vi "Read_Battery_Clear_Fault_VI.vi"() -> ()   [LabVIEW 2017]
uses:
  <vilib>/Plasmionique/MB Master/MB_Master_TCP/MB_Master_TCP.lvclass
  C:/Program Files (x86)/National Instruments/LabVIEW 2017/vi.lib/Plasmionique/MB Master/MB_Master/MB_Master.lvclass
  <vilib>/Plasmionique/MB Master/MB Master.lvlib
panel:
  out "Error?":string
  out "BMS IP Address":string
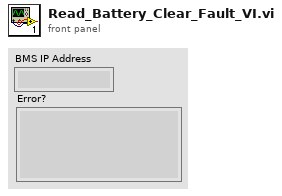
[diagram p1: front panel]
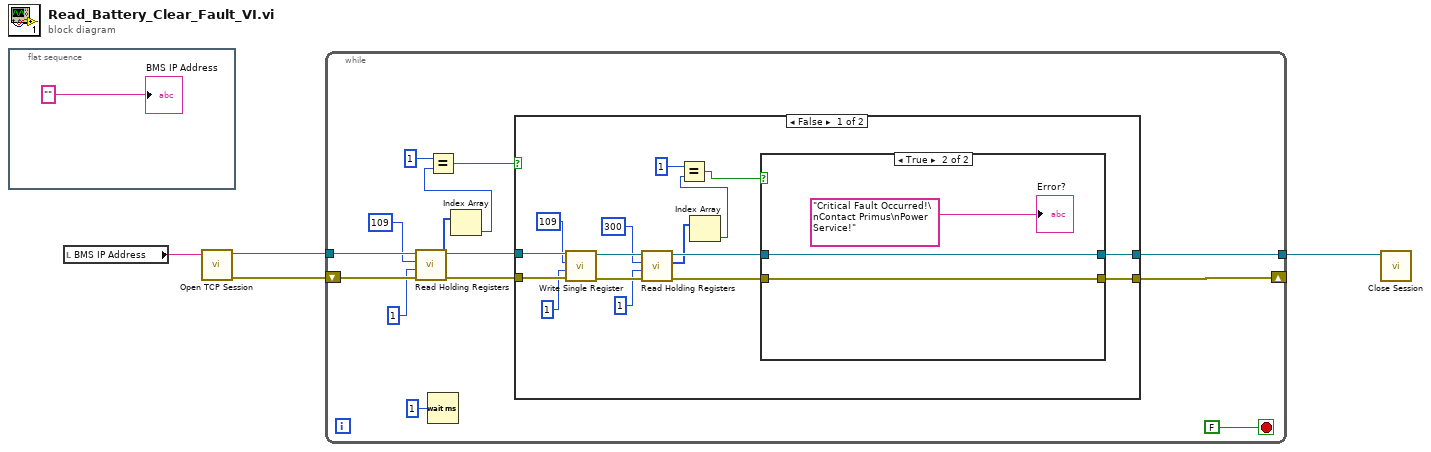
[diagram p0: block diagram]
diagram:
  n1 = flat-sequence {
    frame #0 {
      "BMS IP Address" <- ""
    }
  }
  n2 = local read "BMS IP Address"() -> (w2:string)
  n3 = call <vilib>:"Open TCP Session.vi"("IP Address"=w2) -> ("error out"=w3:errorcluster, "MB_TCP session"=w4:refnum<class "MB_Master_TCP.lvclass">)  [unwired: 9 in]
  n4 = while {
    tunnel: w4 -> [w17]
    shift-right: [w7] -> _
    shift-left: w3 -> [w16]
    tunnel: [w6] -> w1
    stop <- FALSE stop-if-true
    n5 = call <vilib>:"Read Holding Registers.vi"("error in (no error)"=w16, "quantity"=u16 1, "starting address"=u16 109, "MB session in"=w17) -> ("error out"=w12:errorcluster, "Registers"=w11:u16[], "MB session out"=w13:refnum<class "MB_Master_TCP.lvclass">)  [unwired: 5 in]
    n6 = Wait (ms)(milliseconds to wait=u32 1) -> ()  [unwired: 1 out]
    n7 = Index Array(array=w11) -> (element=w10:u16)  [unwired: 1 in]
    n8 = Equal?(x=u16 1, y=w10) -> (x = y?=w8:bool)
    n9 = case shown="False" w8 {
      tunnel: w13 -> [w35 w42]
      tunnel: w12 -> [w34 w41]
      tunnel: [w31 w42] -> w6
      tunnel: [w30 w41] -> w7
      frame False {
        n10 = call <vilib>:"Write Single Register.vi"("error in (no error)"=w34, "value"=u16 1, "address"=u16 109, "MB session in"=w35) -> ("error out"=w28:errorcluster, "MB session out"=w29:refnum<class "MB_Master_TCP.lvclass">)  [unwired: 6 in]
        n11 = call <vilib>:"Read Holding Registers.vi"("error in (no error)"=w28, "quantity"=u16 1, "starting address"=u16 300, "MB session in"=w29) -> ("error out"=w26:errorcluster, "Registers"=w22:u16[], "MB session out"=w27:refnum<class "MB_Master_TCP.lvclass">)  [unwired: 5 in]
        n12 = Index Array(array=w22) -> (element=w23:u16)  [unwired: 1 in]
        n13 = Equal?(x=u16 1, y=w23) -> (x = y?=w21:bool)
        n14 = case shown="True" w21 {
          tunnel: w27 -> [w37 w39]
          tunnel: w26 -> [w36 w38]
          tunnel: [w37 w39] -> w31
          tunnel: [w36 w38] -> w30
          frame False {
          }
          frame True {
            "Error?" <- "Critical Fault Occurred!\nContact Primus\nPower Service!" ("String")
          }
        }
      }
      frame True {
      }
    }
  }
  n15 = call-dynamic "Close Session.vi"("MB TCP session"=w1) -> ()  [unwired: 10 in, 1 out]
